vi "Simple Wrire in TDMS.vi"() -> ()   [LabVIEW 2021]
panel:
  in  "channel name(s) in (Untitled)":string[](array[string])
  in  "group name in (Untitled)":string
  in  "file path":path
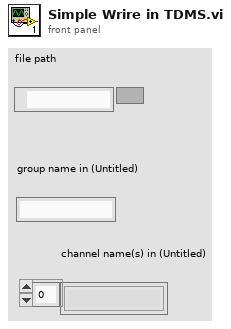
[diagram p1: front panel]
types:
  T1 = enum16{"open", "open or create", "create or replace", "create", "open (read-only)"}
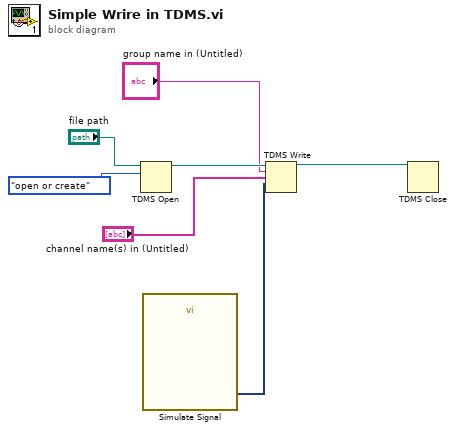
[diagram p0: block diagram]
diagram:
  n1 = TDMS Open(10:T1."open or create" ("operation (0:open)"), 11:"file path") -> (3:w7:refnum<k34>)  [unwired: 5 in, 1 out]
  n2 = call "Simulate Signal"() -> ("Sine with Periodic Noise"=w3:dynamicdata)  [unwired: 14 in, 1 out]
  n3 = TDMS Write(0:w7, 5:"group name in (Untitled)", 7:"channel name(s) in (Untitled)", 9:w3) -> (4:w6:refnum<k34>)  [unwired: 2 in, 3 out]
  n4 = TDMS Close(11:w6) -> ()  [unwired: 1 in, 2 out]
